vi "Query Current.vi"(8 "error in (no error)":errorcluster, 11 "VISA resource name":refnum<visa-resource-name>) -> (0 "error out":errorcluster, 1 "Ch2 Motor current (I)":sgl, 2 "Ch1  Motor current (I)":sgl, 3 "VISA resource name out":refnum<visa-resource-name>, 4 "Ch2 Battery current (I)":sgl, 5 "Motor Currents":T1, 6 "Ch1 Battery current (I)":sgl)   [LabVIEW 2012, in "Roboteq.lvlib"]
uses:
  Roboteq.lvlib
panel:
  out "read buffer 4":string
  out "read buffer 3":string
  out "read buffer 2":string
  out "read buffer":string
  in  "byte count 2":u32
  in  "byte count":u32
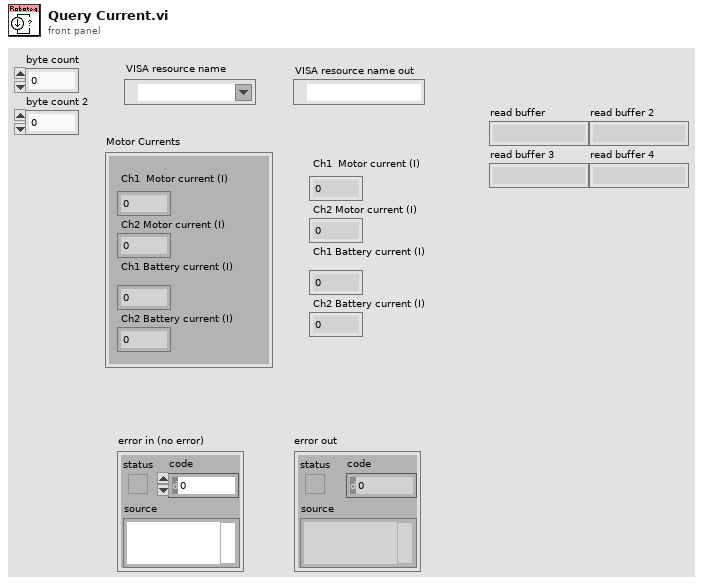
[diagram p1: front panel]
types:
  T1 = cluster{" Ch1  Motor current (I)":sgl, " Ch2 Motor current (I)":sgl, " Ch1 Battery current (I)":sgl, " Ch2 Battery current (I)":sgl}
  T2 = cluster{" Ch1  Motor current (I)":sgl, " Ch2 Motor current (I)":sgl, " Ch1 Battery current (I)":sgl, " Ch2 Battery current (I) 2":sgl}
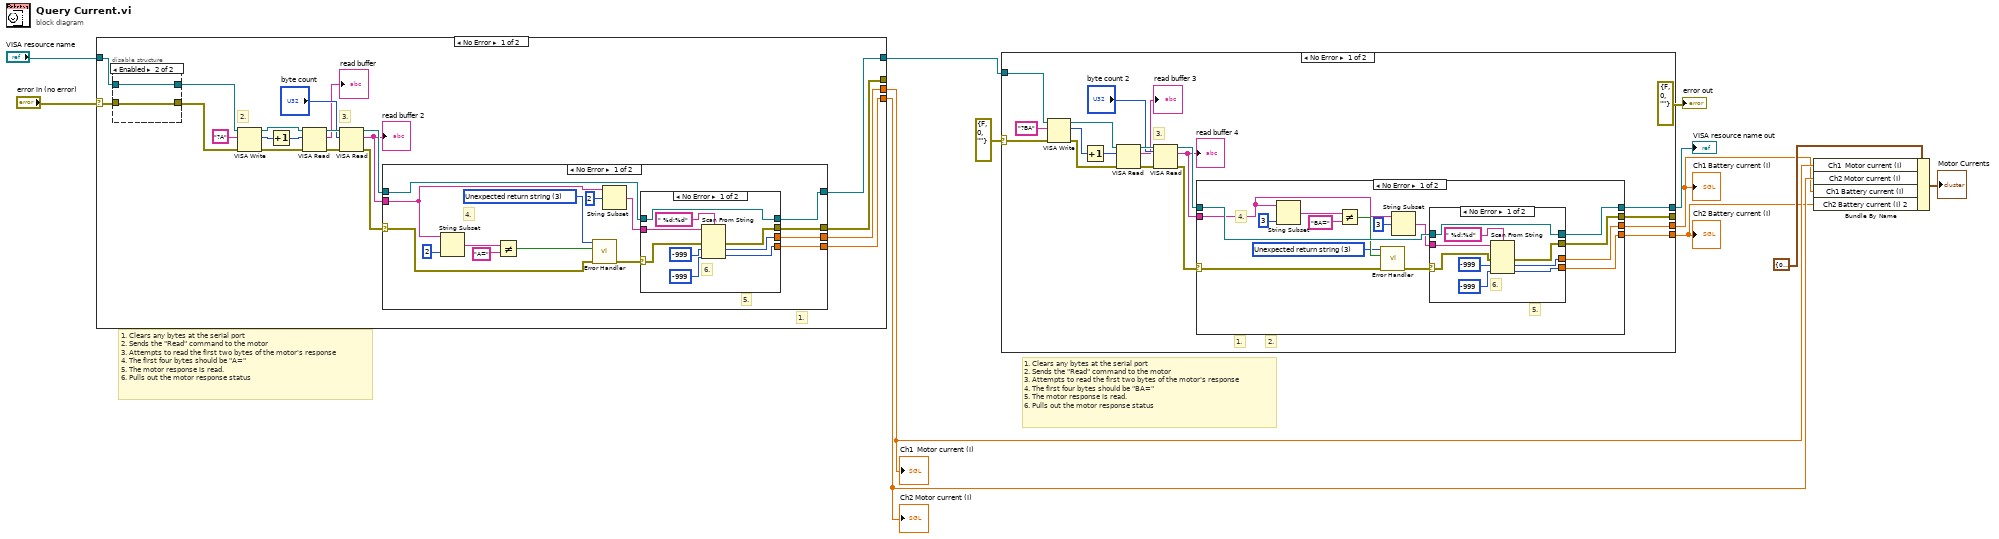
[diagram p0: block diagram]
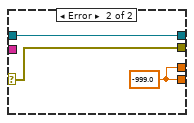
[diagram p2: hidden frame]
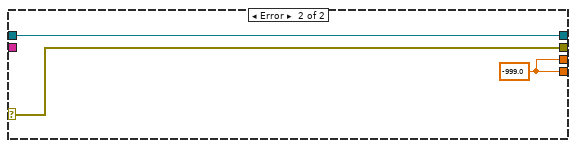
[diagram p3: hidden frame]
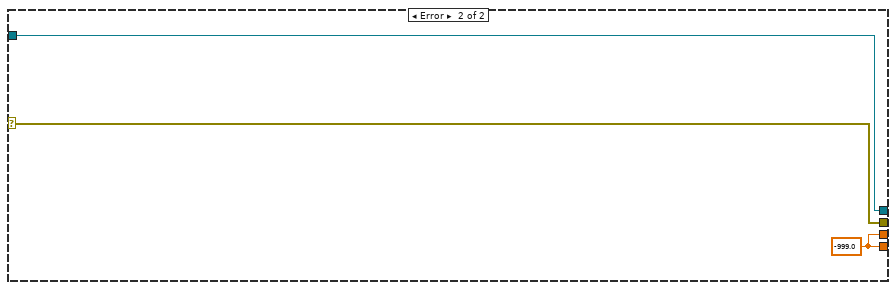
[diagram p4: hidden frame]
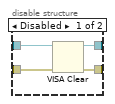
[diagram p5: hidden frame]
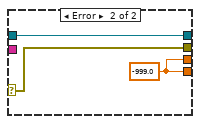
[diagram p6: hidden frame]
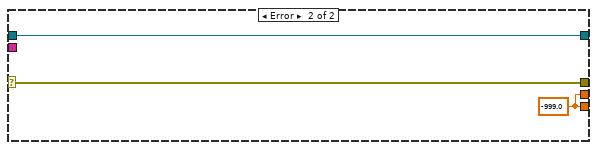
[diagram p7: hidden frame]
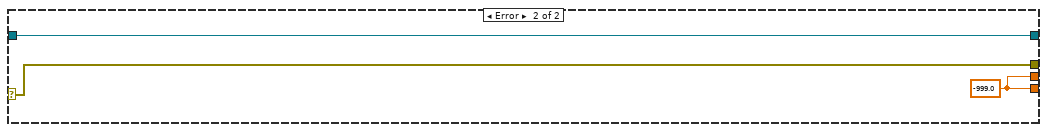
[diagram p8: hidden frame]
diagram:
  # "1. Clears any bytes at the serial port\n2. Sends the \"Read\" command to the motor\n3. Attempts to read the first two bytes of the motor's response\n4. The first four bytes should be \"BA=\"\n5. The motor response is read.\n6. Pulls out the motor response status"
  # "1. Clears any bytes at the serial port\n2. Sends the \"Read\" command to the motor\n3. Attempts to read the first two bytes of the motor's response\n4. The first four bytes should be \"A=\"\n5. The motor response is read.\n6. Pulls out the motor response status"
  n1 = case shown="No Error" "error in (no error)" {
    selector: "error in (no error)" -> [w24 w71]
    tunnel: [w27 w71] -> _
    tunnel: [w28 w70] -> w7
    tunnel: [w29 w70] -> w8
    tunnel: "VISA resource name" -> [w25 w69]
    tunnel: [w26 w69] -> w12
    frame No Error {
      # "1."
      # "3."
      # "2."
      n2 = disable-structure shown="Enabled" {
        disable-tunnel: w25 -> [w33 w38]
        disable-tunnel: w24 -> [w36 w37]
        disable-tunnel: [w35 w38] -> w23
        disable-tunnel: [w34 w37] -> w22
        frame Disabled {
          n3 = VISA Clear(VISA resource name=w33, error in (no error)=w36) -> (VISA resource name out=w35:refnum<visa-resource-name>, error out=w34:errorcluster)
        }
        frame Enabled {
        }
      }
      n4 = VISA Write(VISA resource name=w23, write buffer="?A" ("string"), error in (no error)=w22) -> (VISA resource name out=w20:refnum<visa-resource-name>, return count=w16:u32, error out=w18:errorcluster)
      n5 = Increment(x=w16) -> (x+1=w15:u32)
      n6 = VISA Read(VISA resource name=w20, byte count=w15, error in (no error)=w18) -> (VISA resource name out=w19:refnum<visa-resource-name>, read buffer=→"read buffer":string, error out=w17:errorcluster)  [unwired: 1 out]
      n7 = VISA Read(VISA resource name=w19, byte count="byte count", error in (no error)=w17) -> (VISA resource name out=w31:refnum<visa-resource-name>, read buffer=w30:string, error out=w32:errorcluster)  [unwired: 1 out]
      "read buffer 2" <- w30
      n8 = case shown="No Error" w32 {
        selector: w32 -> [w49 w68]
        tunnel: w30 -> [w41 _]
        tunnel: [w51 w68] -> w27
        tunnel: w31 -> [w53 w67]
        tunnel: [w52 w67] -> w26
        tunnel: [w45 w66] -> w29
        tunnel: [w44 w66] -> w28
        frame No Error {
          w46 = u16 3 items=["Scan timeout"=1, "Invalid motor checksum"=2, "Unexpected return string"=3, "Invalid address range"=4] ("Error type")
          # "5."
          # "4."
          n9 = String Subset(string=w41, length (rest)=2 ("length (rest)")) -> (substring=w42:string)  [unwired: 1 in]
          n10 = Not Equal?(x=w42, y="A=" ("string")) -> (x != y?=w48:bool)
          n11 = call "Error Handler.vi"("error in (no error)"=w49, "Error? (no error)"=w48, "Error type"=w46) -> ("error out"=w50:errorcluster)  [unwired: 8 in]
          n12 = String Subset(string=w41, offset (0)=2 ("length (rest)")) -> (substring=w39:string)  [unwired: 1 in]
          n13 = case shown="No Error" w50 {
            selector: w50 -> [w57 w65]
            tunnel: w39 -> [w58 _]
            tunnel: [w56 w65] -> w51
            tunnel: [w62 w64] -> w52
            tunnel: w53 -> [w62 w64]
            tunnel: [w55 w63] -> w45
            tunnel: [w54 w63] -> w44
            frame No Error {
              # "6."
              n14 = Scan From String(format string=" %d:%d", input string=w58, error in=w57, default 1=-999 ("default value 1"), default 2=-999 ("default value 1")) -> (error out=w56:errorcluster, output 1=w55:i32, output 2=w54:i32)  [unwired: 1 in, 2 out]
            }
            frame Error {
              w63 = sgl -999.0 ("main battery\nvoltage (V)")
            }
          }
        }
        frame Error {
          w66 = sgl -999.0 ("main battery\nvoltage (V)")
        }
      }
    }
    frame Error {
      w70 = sgl -999.0 ("main battery\nvoltage (V)")
    }
  }
  "Ch1  Motor current (I)" <- w8
  "Ch2 Motor current (I)" <- w7
  n15 = case shown="No Error" errorcluster {"status"=FALSE, "code"=0, "source"=""} ("error IO") {
    selector: errorcluster {"status"=FALSE, "code"=0, "source"=""} ("error IO") -> [w81 w122]
    tunnel: [w84 w122] -> _
    tunnel: [w85 w121] -> w5
    tunnel: [w86 w121] -> w6
    tunnel: w12 -> [w82 w120]
    tunnel: [w83 w120] -> w11
    frame No Error {
      # "1."
      # "3."
      # "2."
      n16 = VISA Write(VISA resource name=w82, write buffer="?BA" ("string"), error in (no error)=w81) -> (VISA resource name out=w77:refnum<visa-resource-name>, return count=w79:u32, error out=w74:errorcluster)
      n17 = Increment(x=w79) -> (x+1=w80:u32)
      n18 = VISA Read(VISA resource name=w77, byte count=w80, error in (no error)=w74) -> (VISA resource name out=w76:refnum<visa-resource-name>, read buffer=→"read buffer 3":string, error out=w75:errorcluster)  [unwired: 1 out]
      n19 = VISA Read(VISA resource name=w76, byte count="byte count 2", error in (no error)=w75) -> (VISA resource name out=w88:refnum<visa-resource-name>, read buffer=w87:string, error out=w89:errorcluster)  [unwired: 1 out]
      "read buffer 4" <- w87
      n20 = case shown="No Error" w89 {
        selector: w89 -> [w100 w119]
        tunnel: w87 -> [w92 _]
        tunnel: [w102 w119] -> w84
        tunnel: w88 -> [w104 w118]
        tunnel: [w103 w118] -> w83
        tunnel: [w96 w117] -> w86
        tunnel: [w95 w117] -> w85
        frame No Error {
          w97 = u16 3 items=["Scan timeout"=1, "Invalid motor checksum"=2, "Unexpected return string"=3, "Invalid address range"=4] ("Error type")
          # "5."
          # "4."
          n21 = String Subset(string=w92, length (rest)=3 ("length (rest)")) -> (substring=w93:string)  [unwired: 1 in]
          n22 = Not Equal?(x=w93, y="BA=" ("string")) -> (x != y?=w99:bool)
          n23 = call "Error Handler.vi"("error in (no error)"=w100, "Error? (no error)"=w99, "Error type"=w97) -> ("error out"=w101:errorcluster)  [unwired: 8 in]
          n24 = String Subset(string=w92, offset (0)=3 ("length (rest)")) -> (substring=w90:string)  [unwired: 1 in]
          n25 = case shown="No Error" w101 {
            selector: w101 -> [w108 w116]
            tunnel: w90 -> [w109 _]
            tunnel: [w107 w116] -> w102
            tunnel: [w113 w115] -> w103
            tunnel: w104 -> [w113 w115]
            tunnel: [w106 w114] -> w96
            tunnel: [w105 w114] -> w95
            frame No Error {
              # "6."
              n26 = Scan From String(format string=" %d:%d", input string=w109, error in=w108, default 1=-999 ("default value 1"), default 2=-999 ("default value 1")) -> (error out=w107:errorcluster, output 1=w106:i32, output 2=w105:i32)  [unwired: 1 in, 2 out]
            }
            frame Error {
              w114 = sgl -999.0 ("main battery\nvoltage (V)")
            }
          }
        }
        frame Error {
          w117 = sgl -999.0 ("main battery\nvoltage (V)")
        }
      }
    }
    frame Error {
      w121 = sgl -999.0 ("main battery\nvoltage (V)")
    }
  }
  "VISA resource name out" <- w11
  "Ch2 Battery current (I)" <- w5
  "Ch1 Battery current (I)" <- w6
  n27 = Bundle By Name(cluster=T2 {" Ch1  Motor current (I)"=0.0, " Ch2 Motor current (I)"=0.0, " Ch1 Battery current (I)"=0.0, " Ch2 Battery current (I) 2"=0.0} ("Motor Currents"), "Ch1  Motor current (I)"=w8, "Ch2 Motor current (I)"=w7, "Ch1 Battery current (I)"=w6, "Ch2 Battery current (I) 2"=w5) -> (→"Motor Currents":T2)
  "error out" <- errorcluster {"status"=FALSE, "code"=0, "source"=""} ("error out")
